vi "FlashLamp_OFF VI.vi"(1 "Error In":errorcluster caption="Fehler (Eingang, kein Fehler)") -> (0 "error out":errorcluster)   [LabVIEW 2016]
uses:
  Utility/Global_Laser.vi
  Program Files (x86)/OPOTEK_DLL/OPOTEK.dll
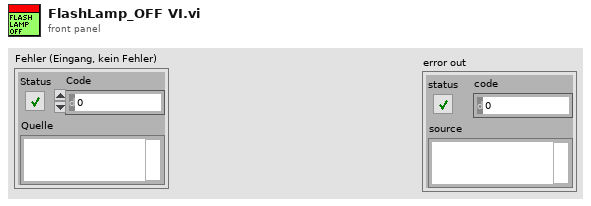
[diagram p1: front panel]
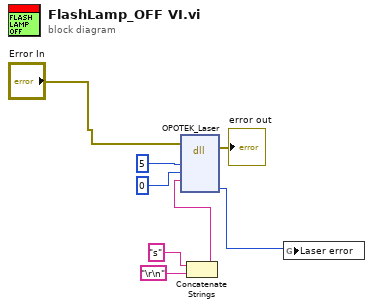
[diagram p0: block diagram]
diagram:
  n1 = Concatenate Strings("s", "\r\n") -> (w4:string)
  n2 = dll-call lib="C:/Program Files (x86)/OPOTEK_DLL/OPOTEK.dll" fn="OPOTEK_Laser"(error in="Error In", "action"=i8 5, "parameter"=i16 0, "stringToSend"=w4) -> (error out=→"error out":errorcluster, "error_Code"=w1:i32)  [unwired: 7 in, 1 out]
  n3 = global write "Global_Laser.vi" "Laser error"(w1) -> ()
